vi "Core Write DAQ DVR FIFO.vi"(6 "FIFO Timestamps":T1, 8 "error in (no error)":errorcluster, 9 "Timeout (ms)":i32=100, 10 "Data In":refnum<data-value>[](array[refnum]), 11 "CIFTag in":refnum<class "CIF_NIChn_Fifo_DAQ.lvclass">) -> (0 "error out":errorcluster, 1 "timed out?":bool, 2 "Data Out":refnum<data-value>[](array[refnum]), 3 "CIFTag out":refnum<class "CIF_NIChn_Fifo_DAQ.lvclass">)   [LabVIEW 2021, in "CIF_NIChn_Fifo_DAQ.lvclass"]
uses:
  CIF_NIChn_Fifo_DAQ.lvclass
  NIChn/CIF_NIChn.lvclass
  D:/dev/Packages/Channel_Manager/src/CIF_NIChn/NIChn/CIF_NIChn.lvclass
  <vilib>/CIF Foundation/CIF Channels/CIFChannels/CIFChannelCore.lvlib
  ChannelCommon/typedef/TimeStamps.ctl
  ChannelCommon/ChannelCommon.lvlib
  ChannelCommon/typedef/Datatype Waveform.ctl
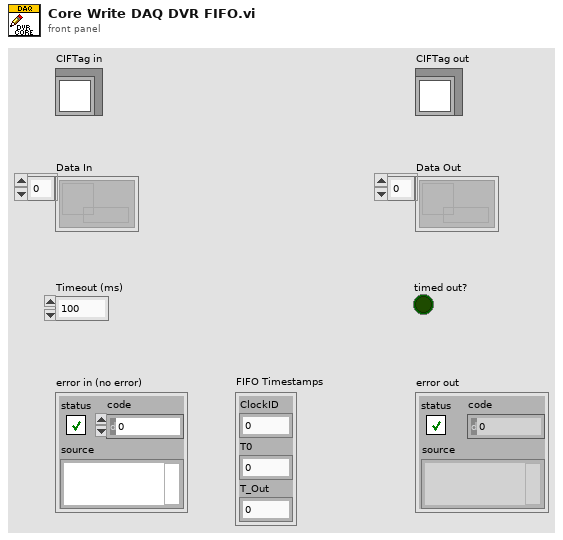
[diagram p1: front panel]
types:
  T1 = typedef "ChannelCommon.lvlib/TimeStamps.ctl" = cluster{"ClockID":u8, "T0":i64, "T_Out":i64}
  T2 = typedef "ChannelCommon.lvlib/FIFO Header.ctl" = cluster{"Length":u64, "T0":i64, "T_Out":i64, "T_Tx":i64, "Ctr":u64, "ClockID":u8}
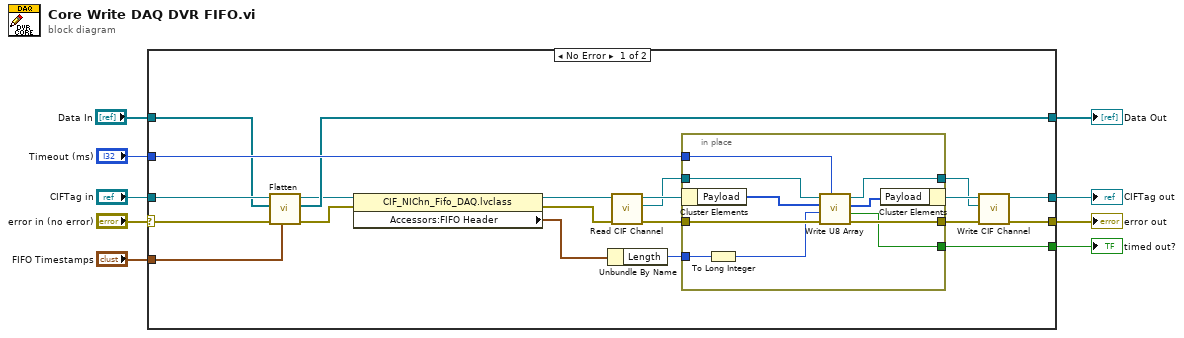
[diagram p0: block diagram]
diagram:
  n1 = case shown="No Error" "error in (no error)" {
    selector: "error in (no error)" -> [w25 w43]
    tunnel: [w27 w43] -> w8
    tunnel: [w29 w42] -> w6
    tunnel: "CIFTag in" -> [w26 w42]
    tunnel: [w30 _] -> w5
    tunnel: "Timeout (ms)" -> [w28 _]
    tunnel: [w24 w41] -> w1
    tunnel: "Data In" -> [w23 w41]
    tunnel: "FIFO Timestamps" -> [w22 _]
    frame No Error {
      n2 = call "Flatten.vi"("FIFO Timestamps"=w22, "error in (no error)"=w25, "Data In"=w23, "CIFTag in"=w26) -> ("error out"=w15:errorcluster, "Data Out"=w24:refnum<data-value>[], "CIFTag out"=w14:refnum<class "CIF_NIChn_Fifo_DAQ.lvclass">)  [unwired: 5 in]
      n3 = property class="CIF_NIChn_Fifo_DAQ.lvclass"(reference=w14, error in=w15) -> (reference out=w13:refnum<class "CIF_NIChn_Fifo_DAQ.lvclass">, error out=w10:errorcluster, "Accessors:FIFO Header"=w12:T2)
      n4 = Unbundle By Name(w12) -> ("Length"=w11:u64)
      n5 = call "Read CIF Channel.vi"("error in (no error)"=w10, "CIFTag in"=w13) -> ("error out"=w20:errorcluster, "CIF Channel"=w17:refnum<k21>, "CIFTag out"=w21:refnum<class "CIF_NIChn_Fifo_DAQ.lvclass">)  [unwired: 7 in]
      n6 = in-place {
        in-place-border: w20 -> [w40]
        in-place-border: [w39] -> w18
        in-place-border: [w38] -> w30
        in-place-border: w17 -> [w37]
        in-place-border: [w36] -> w16
        in-place-border: w28 -> [w35]
        in-place-border: w11 -> [w33]
        n7 = in-place-cluster #1(w21) -> ("Payload"=w34:u8[])
        n8 = To Long Integer(number=w33) -> (32bit integer=w31:i32)
        n9 = call <vilib>:"Write U8 Array.vi"("Timeout (ms)"=w35, "error in"=w40, "Number of Elements"=w31, "U8 Array in"=w34, "CIF Channel in"=w37) -> ("error out"=w39:errorcluster, "Timed out?"=w38:bool, "U8 Array out"=w32:u8[], "CIF Channel out"=w36:refnum<k21>)  [unwired: 3 in]
        n10 = in-place-cluster #1("Payload"=w32) -> (w19:refnum<class "CIF_NIChn_Fifo_DAQ.lvclass">)
      }
      n11 = call "Write CIF Channel.vi"("error in (no error)"=w18, "CIF Channel"=w16, "CIFTag in"=w19) -> ("error out"=w27:errorcluster, "CIFTag out"=w29:refnum<class "CIF_NIChn_Fifo_DAQ.lvclass">)  [unwired: 7 in]
    }
    frame Error {
    }
  }
  "error out" <- w8
  "CIFTag out" <- w6
  "timed out?" <- w5
  "Data Out" <- w1
